vi "FTW-SQLite-OpenConnection-Path.vi"(5 "Database Filepath":path, 7 "Access Mode":T1, 11 "error in":errorcluster) -> (4 "SQLite Connection":refnum<data-value>, 15 "error out":errorcluster)   [LabVIEW 2015]
uses:
  core/FTW-SQLite-Core-Structure.ctl
  core/FTW-SQLite-Core-AccessMode.ctl
  core/FTW-SQLite-Core-DatabaseType.ctl
panel:
  # "Inputs"
  # "Outputs"
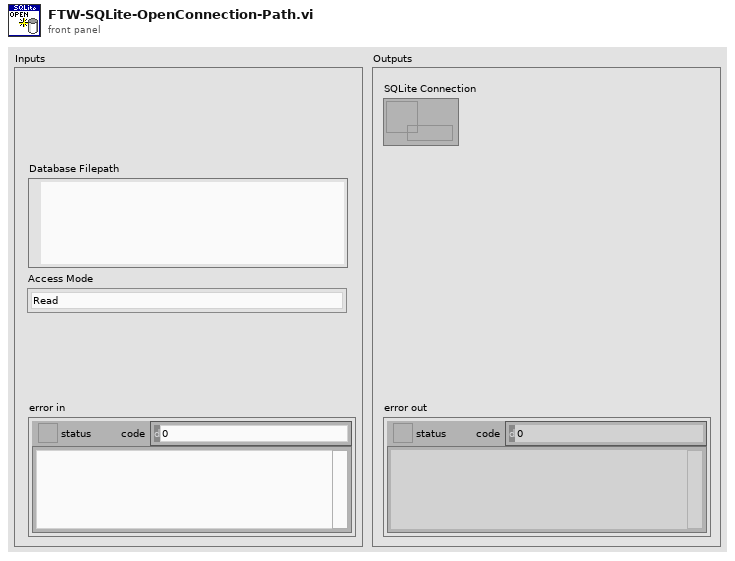
[diagram p1: front panel]
types:
  T1 = typedef "FTW-SQLite-Core-AccessMode.ctl" = enum16{"Read", "Read/Write", "Read/Write/Create"}
  T2 = typedef "FTW-SQLite-Core-DatabaseType.ctl" = enum16{"Disk", "Memory"}
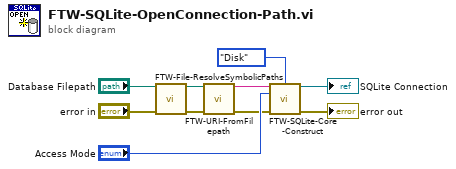
[diagram p0: block diagram]
diagram:
  n1 = call "FTW-File-ResolveSymbolicPaths.vi"("Unresolved Path"="Database Filepath", "error in"="error in") -> ("Resolved Path"=w3:path, "error out"=w1:errorcluster)  [unwired: 12 in]
  n2 = call "FTW-URI-FromFilepath.vi"("Path"=w3, "error in"=w1) -> ("URI"=w6:string, "error out"=w7:errorcluster)  [unwired: 12 in]
  n3 = call "FTW-SQLite-Core-Construct.vi"("Database URI"=w6, "Database Type"=FTW-SQLite-Core-DatabaseType."Disk", "Access Mode"="Access Mode", "error in"=w7) -> ("SQLite Connection"=→"SQLite Connection":refnum<data-value>, "error out"=→"error out":errorcluster)  [unwired: 9 in, 1 out]
